vi "dvp Vi Get Strobe Output Type.vi"(10 "pStrobeOutputType":u32(ring) items=["STROBE_OUT_OFF", "STROBE_OUT_LOW", "STROBE_OUT_HIGH"], 11 "handle":u32) -> (2 "pStrobeOutputType out":u32(ring) items=["STROBE_OUT_OFF", "STROBE_OUT_LOW", "STROBE_OUT_HIGH"], 3 "function return":u32(ring))   [LabVIEW 2018, in "LabViewDVPCamera.lvlib"]
doc: "LabviewDvp2Api dvpStatus dvpViGetStrobeOutputType(dvpHandle handle, dvpStrobeOutputType *pStrobeOutputType);"
uses:
  LabViewDVPCamera.lvlib
  LabViewDVPCamera/LabViewDVPCamera.dll
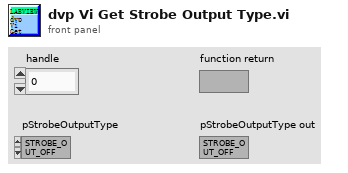
[diagram p1: front panel]
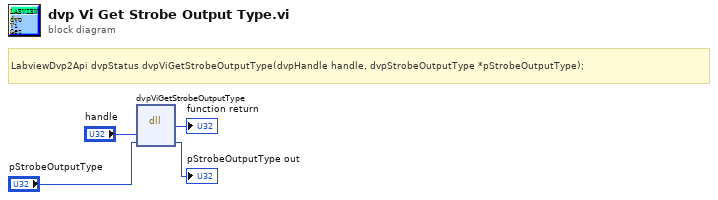
[diagram p0: block diagram]
diagram:
  # "LabviewDvp2Api dvpStatus dvpViGetStrobeOutputType(dvpHandle handle, dvpStrobeOutputType *pStrobeOutputType);"
  n1 = dll-call lib="C:/Program Files (x86)/DVP2 Labview cn 64/Sample/LabViewDVPCamera/LabViewDVPCamera.*" fn="dvpViGetStrobeOutputType"("handle"="handle", "pStrobeOutputType"="pStrobeOutputType") -> (→"function return":u32, "pStrobeOutputType"=→"pStrobeOutputType out":u32)  [unwired: 4 in, 2 out]
